vi "Get Sub Panel.vi"(8 "error in (no error)":errorcluster, 11 "Monedas in":refnum<class "Monedas.lvclass">) -> (0 "error out":errorcluster, 2 "Sub Panel":refnum<vi>, 3 "Monedas out":refnum<class "Monedas.lvclass">)   [LabVIEW 2021, in "Monedas.lvlib" / "Monedas.lvclass"]
uses:
  Monedas.lvclass
  Monedas.lvclass/Monedas.ctl
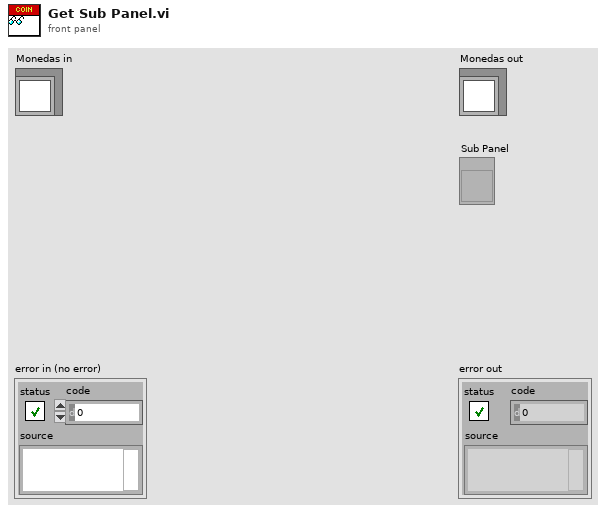
[diagram p1: front panel]
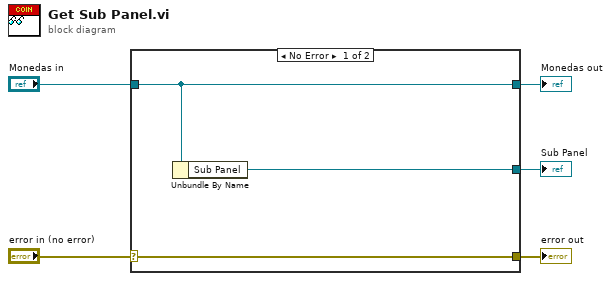
[diagram p0: block diagram]
diagram:
  n1 = case shown="No Error" "error in (no error)" {
    selector: "error in (no error)" -> [w8 w9]
    tunnel: [w8 w9] -> w4
    tunnel: [w7 w10] -> w2
    tunnel: "Monedas in" -> [w7 w10]
    tunnel: [w6 _] -> w1
    frame No Error {
      n2 = Unbundle By Name(w7) -> ("Sub Panel"=w6:refnum<vi>)
    }
    frame Error {
    }
  }
  "error out" <- w4
  "Monedas out" <- w2
  "Sub Panel" <- w1
